vi "TDelay.vi"(8 "Error in":errorcluster, 9 "delay":i32=1, 10 "input":dbl) -> (0 "Error out":errorcluster, 2 "output":dbl)   [LabVIEW 2022 SP3]
uses:
  <vilib>/addons/Digital Filter Design/Process.llb/DFD Integer Delay (PtByPt).vi
  <vilib>/addons/Digital Filter Design/NI_DigFilterLicensed.lvlib
panel:
  out "Error Message":string
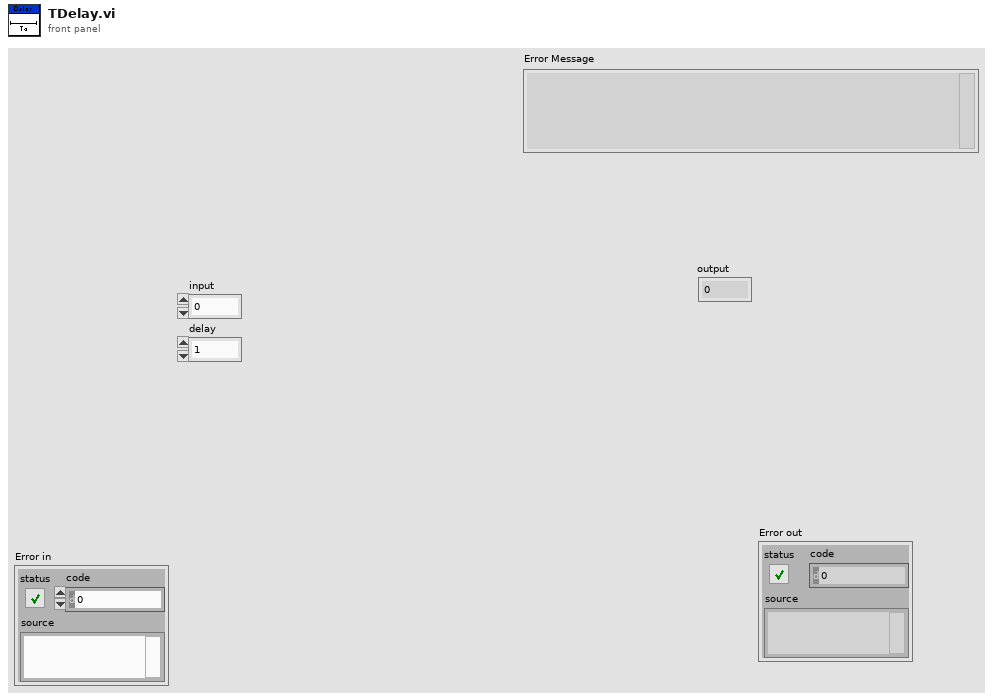
[diagram p1: front panel]
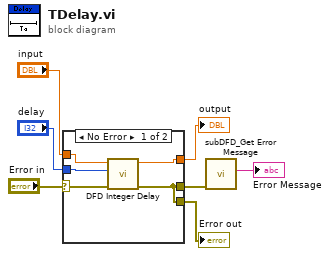
[diagram p0: block diagram]
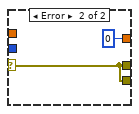
[diagram p2: hidden frame]
diagram:
  n1 = case shown="No Error" "Error in" {
    selector: "Error in" -> [w10 w14]
    tunnel: [w9 w14] -> w7
    tunnel: "input" -> [w11 _]
    tunnel: "delay" -> [w12 _]
    tunnel: [w9 w14] -> w2
    tunnel: [w8 0 ("input")] -> w1
    frame No Error {
      n2 = call-poly <vilib>:"DFD Integer Delay.vi"("error in (no error)"=w10, "delay"=w12, "signal in"=w11) -> ("error out"=w9:errorcluster, "signal out"=w8:dbl)  [unwired: 1 in, 6 out]
    }
    frame Error {
    }
  }
  "Error out" <- w7
  "output" <- w1
  n3 = call <vilib>:"subDFD_Get Error Message.vi"("error in (no error)"=w2) -> ("Error Message"=→"Error Message":string)  [unwired: 10 out]
